vi "grSim_RobotReplacement Encoder.vi"(10 "Robot":T1) -> (2 "Array out":u8[](array[numeric]))   [LabVIEW 2022 SP3, in "Communication.lvclass"]
uses:
  Communication.lvclass
  Paths/grSim Packet Command UDP Test Folder/grSim/grSim RobotReplacement.ctl
panel:
  out "Communication out":refnum<class "Communication.lvclass">
  in  "Communication in":refnum<class "Communication.lvclass">
  out "error out":errorcluster
  in  "error in (no error)":errorcluster
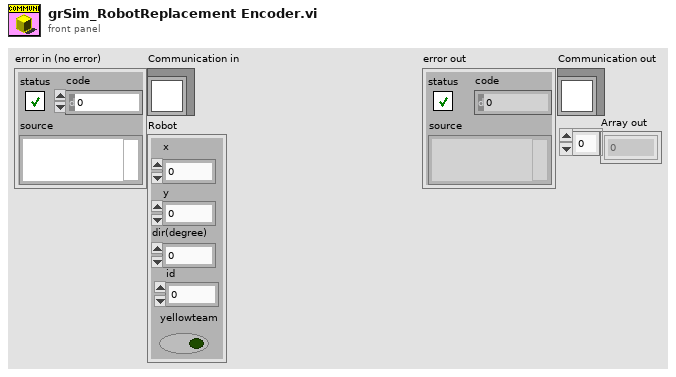
[diagram p1: front panel]
types:
  T1 = typedef "grSim RobotReplacement.ctl" = cluster{"x":dbl, "y":dbl, "dir(degree)":dbl, "yellowteam":bool, "id":u32}
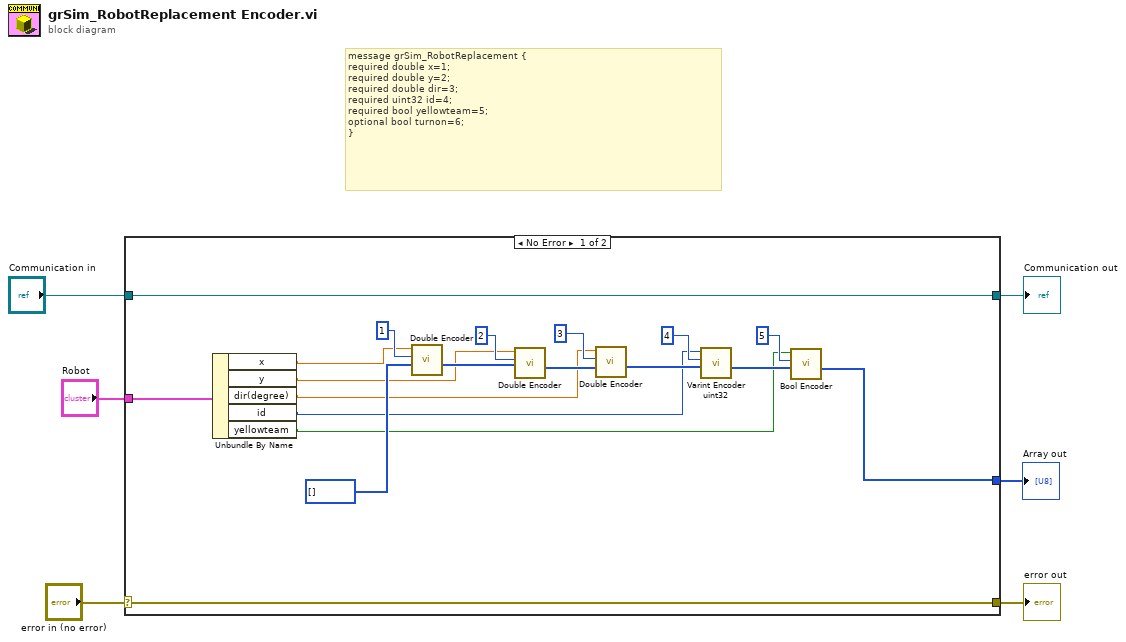
[diagram p0: block diagram]
diagram:
  # "message grSim_RobotReplacement {\nrequired double x=1;\nrequired double y=2;\nrequired double dir=3;\nrequired uint32 id=4;\nrequired bool yellowteam=5;\noptional bool turnon=6;\n}"
  n1 = case shown="No Error" "error in (no error)" {
    selector: "error in (no error)" -> [w24 w27]
    tunnel: [w24 w27] -> w5
    tunnel: [w25 w26] -> w3
    tunnel: "Communication in" -> [w25 w26]
    tunnel: [w13 _] -> w2
    tunnel: "Robot" -> [w12 _]
    frame No Error {
      n2 = Unbundle By Name(w12) -> ("x"=w7:dbl, "y"=w8:dbl, "dir(degree)"=w9:dbl, "id"=w10:u32, "yellowteam"=w11:bool)
      n3 = call "Double Encoder.vi"("Array In"=u8[] [] ("Array in"), "Key"=1, "Value"=w7) -> ("Array"=w18:u8[])  [unwired: 8 in]
      n4 = call "Double Encoder.vi"("Array In"=w18, "Key"=2, "Value"=w8) -> ("Array"=w17:u8[])  [unwired: 8 in]
      n5 = call "Double Encoder.vi"("Array In"=w17, "Key"=3, "Value"=w9) -> ("Array"=w16:u8[])  [unwired: 8 in]
      n6 = call "Varint Encoder uint32.vi"("Array In"=w16, "Key"=4, "Value"=w10) -> ("Array"=w15:u8[])  [unwired: 8 in]
      n7 = call "Bool Encoder.vi"("Array In"=w15, "Key"=5, "Value"=w11) -> ("Array"=w13:u8[])  [unwired: 8 in]
    }
    frame Error {
    }
  }
  "error out" <- w5
  "Communication out" <- w3
  "Array out" <- w2
